vi "UDP Data Link Initialization VI.vi"(8 "error in (no error)":errorcluster, 10 "Custom XML":string, 11 "Device Item Ref in":T1 format="%.0x") -> (0 "error out":errorcluster, 3 "Device Item Ref out":T1 format="%.0x")   [LabVIEW 2012, in "UDP Data Link System Explorer.lvlib"]
uses:
  UDP Data Link System Explorer.lvlib
  <vilib>/NI Veristand/Custom Device API/Custom Device Item Ref.ctl
  <vilib>/NI Veristand/Custom Device API/Custom Device API.lvlib
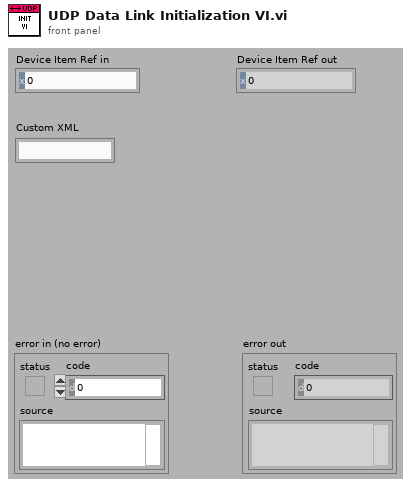
[diagram p1: front panel]
types:
  T1 = typedef "Custom Device API.lvlib/Custom Device Item Ref.ctl" = u64
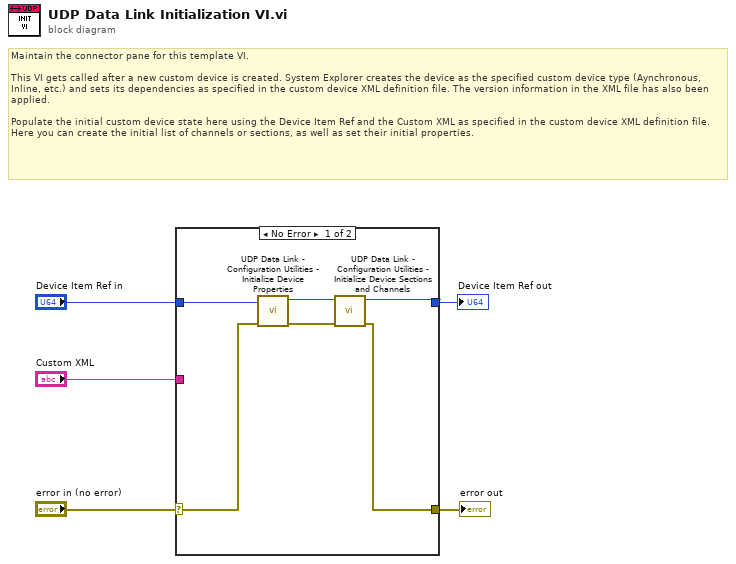
[diagram p0: block diagram]
diagram:
  # "Maintain the connector pane for this template VI.\n\nThis VI gets called after a new custom device is created. System Explorer creates the device as the specified custom device type (Aynchronous, Inline, etc.) and sets its dependencies as specified in the custom device XML definition file. The version information in the XML file has also been applied.\n\nPopulate the initial custom device state here using the Device Item Ref and the Custom XML as specified in the custom device XML definition file. Here you can create the initial list of channels or sections, as well as set their initial properties."
  n1 = case shown="No Error" "error in (no error)" {
    selector: "error in (no error)" -> [w10 w13]
    tunnel: [w7 w13] -> w5
    tunnel: [w6 w12] -> w3
    tunnel: "Device Item Ref in" -> [w11 w12]
    tunnel: "Custom XML" -> [_ _]
    frame No Error {
      n2 = call "UDP Data Link - Configuration Utilities - Initialize Device Properties.vi"("error in (no error)"=w10, "Device Item Ref in"=w11) -> ("error out"=w8:errorcluster, "Item Ref out"=w9:T1)  [unwired: 8 in]
      n3 = call "UDP Data Link - Configuration Utilities - Initialize Device Sections and Channels.vi"("error in (no error)"=w8, "Item Ref out"=w9) -> ("error out"=w7:errorcluster, "Parent Ref out"=w6:T1)  [unwired: 8 in]
    }
    frame Error {
    }
  }
  "error out" <- w5
  "Device Item Ref out" <- w3
